vi "RemoveEmptyLinesFromControlFile.vi"(8 "Error In":errorcluster, 11 "Control File Path":path) -> (0 "Error Out":errorcluster)   [LabVIEW 2019, in "CEPM.lvlib"]
uses:
  CEPM.lvlib
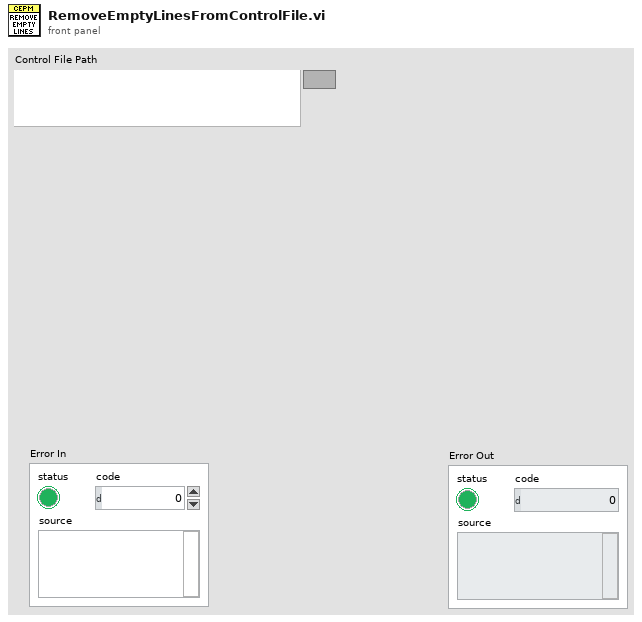
[diagram p1: front panel]
types:
  T1 = enum16{"open", "replace", "create", "open or create", "replace or create", "replace or create with confirmation"}
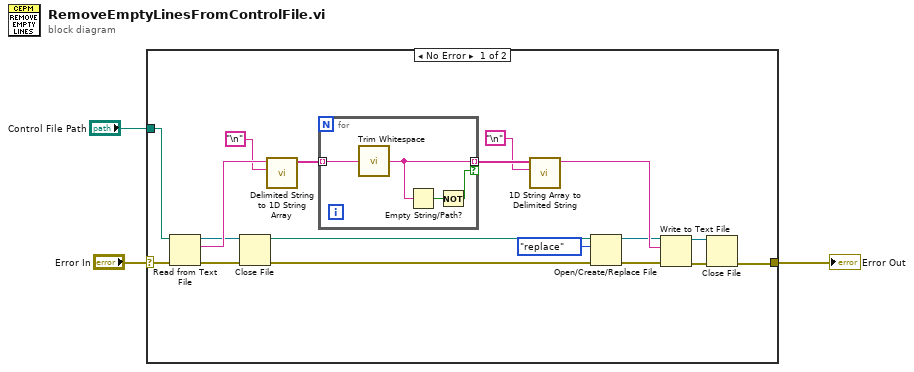
[diagram p0: block diagram]
diagram:
  n1 = case shown="No Error" "Error In" {
    selector: "Error In" -> [w13 w26]
    tunnel: [w14 w26] -> w2
    tunnel: "Control File Path" -> [w12 _]
    frame No Error {
      n2 = Read from Text File(file (use dialog)=w12, error in=w13) -> (refnum out=w10:refnum<file>, text=w21:string, error out=w17:errorcluster)  [unwired: 2 in, 1 out]
      n3 = Close File(refnum=w10, error in=w17) -> (path=w8:path, error out=w11:errorcluster)
      n4 = call <vilib>:"Delimited String to 1D String Array.vi"("delimiter"="\n", "delimited string"=w21) -> ("string array"=w20:string[])  [unwired: 9 in]
      n5 = for {
        tunnel: w20 -> [w25] mode=indexing
        tunnel: [w24] -> w19 mode=indexing if=w22
        n6 = call <vilib>:"Trim Whitespace.vi"("string"=w25) -> ("trimmed string"=w24:string)  [unwired: 1 in]
        n7 = Empty String/Path?(string/path=w24) -> (empty?=w23:bool)
        n8 = Not(x=w23) -> (.not. x?=w22:bool)
      }
      n9 = call <vilib>:"1D String Array to Delimited String.vi"("delimiter"="\n", "string array"=w19) -> ("delimited string"=w18:string)  [unwired: 9 in]
      n10 = Open/Create/Replace File(file path (use dialog)=w8, error in=w11, operation (0:open)=T1."replace") -> (refnum out=w7:refnum<file>, error out=w9:errorcluster)  [unwired: 3 in, 1 out]
      n11 = Write to Text File(file (use dialog)=w7, text=w18, error in=w9) -> (refnum out=w15:refnum<file>, error out=w16:errorcluster)  [unwired: 1 in, 1 out]
      n12 = Close File(refnum=w15, error in=w16) -> (error out=w14:errorcluster)  [unwired: 1 out]
    }
    frame Error {
    }
  }
  "Error Out" <- w2
